vi "Griddy Reserve.vi"   [LabVIEW 2020]
uses:
  manipulator/Implementation/Typedefs/Teleop Manipulator Commands.ctl
types:
  T1 = typedef "Teleop Manipulator Commands.ctl" = enum16{"idle", "intake cone", "intake cube", "score low cone", "score low cube", "score mid cone", "score mid cube", "score high cone", "score high cube"}
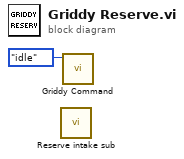
[diagram p0: block diagram]
diagram:
  n1 = call "Reserve intake sub.vi"() -> ()  [unwired: 11 in, 1 out]
  n2 = call "Griddy Command.vi"("Griddy Command"=Teleop_Manipulator_Commands."idle") -> ()  [unwired: 10 in, 1 out]
